vi "resize.vi"(8 "error in (no error)":errorcluster, 11 "HGF_Rendezvous":refnum<class "HGF_Rendezvous.lvclass">) -> (0 "error out":errorcluster, 3 "dup HGF_Rendezvous":refnum<class "HGF_Rendezvous.lvclass">)   [LabVIEW 2014, in "HGF_BaseClasses.lvlib" / "HGF_Rendezvous.lvclass"]
doc: "Resize rendezvous."
uses:
  HGF_Rendezvous.lvclass
  HGF_Auxiliary/HGF_Auxiliary.lvlib
  HGF_Auxiliary/Severity.ctl
  HGF_Auxiliary/ErrorCode.ctl
panel:
  out "new size":i32
  in  "size change (0)":i32
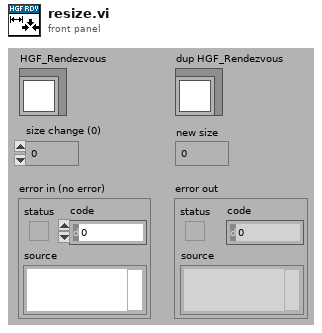
[diagram p1: front panel]
types:
  T1 = typedef "HGF_Auxiliary.lvlib/ErrorCode.ctl" = enum32{"No error", "Function not supported.", "This VI is for friends only.", "Reference object aready exisits.", "Parameter out of range.", "Not a rendezvous.", "Invalid notifier reference.", "Invalid queue reference.", "Self-Test not supported.", "Reset not supported.", "IDN query not supported.", "Error query not supported.", "Incorrect addressee.", "Object already exists.", "No class name specified", "Driver not supported", "Attribute is not writable"}
  T2 = typedef "HGF_Auxiliary.lvlib/Severity.ctl" = enum16{"Info", "Warning", "Fault", "Error", "Fatal"}
  T3 = typedef "Rendezvous RefNum" = refnum<k1>
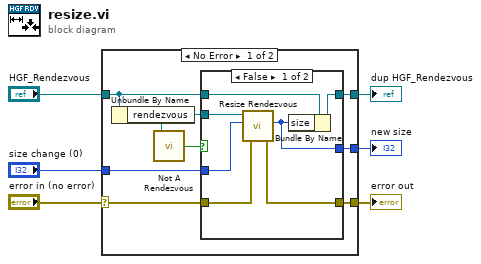
[diagram p0: block diagram]
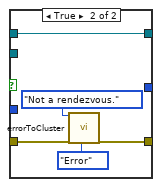
[diagram p2: hidden frame]
diagram:
  n1 = case shown="No Error" "error in (no error)" {
    selector: "error in (no error)" -> [w12 w28]
    tunnel: [w13 w28] -> w5
    tunnel: [w9 w27] -> w3
    tunnel: "HGF_Rendezvous" -> [w8 w27]
    tunnel: "size change (0)" -> [w10 _]
    tunnel: [w7 _] -> w1
    frame No Error {
      n2 = Unbundle By Name(w8) -> ("rendezvous"=w11:T3)
      n3 = call <vilib>:"Not A Rendezvous.vi"("rendezvous"=w11) -> ("not a rendezvous"=w14:bool)
      n4 = case shown="False" w14 {
        tunnel: [w16 w24] -> w13
        tunnel: w12 -> [w17 w25]
        tunnel: w11 -> [w21 _]
        tunnel: w10 -> [w20 _]
        tunnel: [w18 w26] -> w9
        tunnel: w8 -> [w19 w26]
        tunnel: [w15 _] -> w7
        frame False {
          n5 = call <vilib>:"Resize Rendezvous.vi"("error in (no error)"=w17, "size change (0)"=w20, "rendezvous"=w21) -> ("error out"=w16:errorcluster, "new size"=w15:i32)  [unwired: 3 out]
          n6 = Bundle By Name(cluster=w19, "size"=w15) -> (w18:refnum<class "HGF_Rendezvous.lvclass">)
        }
        frame True {
          n7 = call "errorToCluster.vi"("error code"=ErrorCode."Not a rendezvous.", "error in (no error)"=w25, "severity (Error)"=Severity."Error") -> ("error out"=w24:errorcluster)  [unwired: 2 in, 14 out]
        }
      }
    }
    frame Error {
    }
  }
  "error out" <- w5
  "dup HGF_Rendezvous" <- w3
  "new size" <- w1
